vi "Read Waveform Measurement (Px).vi"(0 "VISA resource name":refnum<visa-resource-name>, 5 "Parameter (0: P1)":u16(ring) items=["P1", "P2", "P3", "P4", "P5"], 11 "error in (no error)":errorcluster) -> (4 "VISA resource name out":refnum<visa-resource-name>, 6 "Value":dbl format="%#_3f", 15 "error out":errorcluster)   [LabVIEW 2021, in "Siglent SDS 1000 2000 Series.lvlib"]
doc: "Reads a result of the parameter measured on P1 through P5 and returns the status. Note that for multi-valued parameters (parameters that can return more than 1 value per sweep) the value is the last measured event, and not the average over the entire waveform. Attempting to read back a non-existent parameter will result in an unresolved parsing error from the instrument."
uses:
  <instrlib>/Siglent SDS 1000 2000 Series/Siglent SDS 1000 2000 Series.lvlib
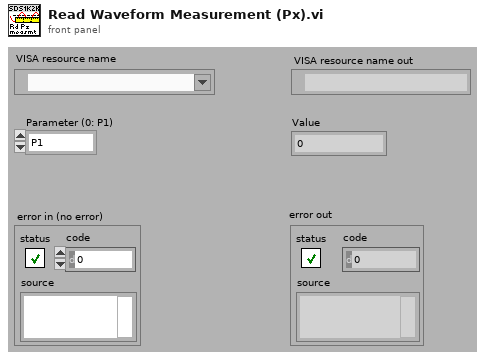
[diagram p1: front panel]
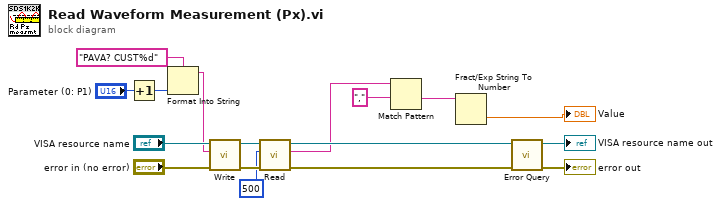
[diagram p0: block diagram]
diagram:
  n1 = Increment(x="Parameter (0: P1)") -> (x+1=w6:u16)
  n2 = Format Into String(format string="PAVA? CUST%d", w6) -> (resulting string=w8:string)  [unwired: 2 in, 1 out]
  n3 = call <instrlib>:"Write.vi"("error in (no error)"="error in (no error)", "Write Buffer"=w8, "VISA resource name"="VISA resource name") -> ("error out"=w13:errorcluster, "VISA resource name out"=w14:refnum<visa-resource-name>)  [unwired: 6 in, 1 out]
  n4 = call <instrlib>:"Read.vi"("error in (no error)"=w13, "Byte Count"=u32 500, "VISA resource name"=w14) -> ("error out"=w1:errorcluster, "Read Buffer"=w5:string, "VISA resource name out"=w11:refnum<visa-resource-name>)  [unwired: 5 in, 1 out]
  n5 = Match Pattern(string=w5, regular expression=",") -> (after substring=w3:string)  [unwired: 1 in, 3 out]
  n6 = Fract/Exp String To Number(string=w3) -> (number=→"Value":dbl)  [unwired: 3 in, 1 out]
  n7 = call <instrlib>:"Error Query.vi"("error in (no error)"=w1, "VISA resource name"=w11) -> ("error out"=→"error out":errorcluster, "VISA resource name out"=→"VISA resource name out":refnum<visa-resource-name>)  [unwired: 6 in, 2 out]
